vi "Get Variant Attributes.vi"(8 "错误输入":errorcluster, 11 "Variant":variant) -> (0 "错误输出":errorcluster, 1 "Values":variant[](array[variant]), 2 "Names":string[](array[string]), 3 "dup Variant":variant)   [LabVIEW 2012, in "TD Tools.lvlib"]
uses:
  TD Tools.lvlib
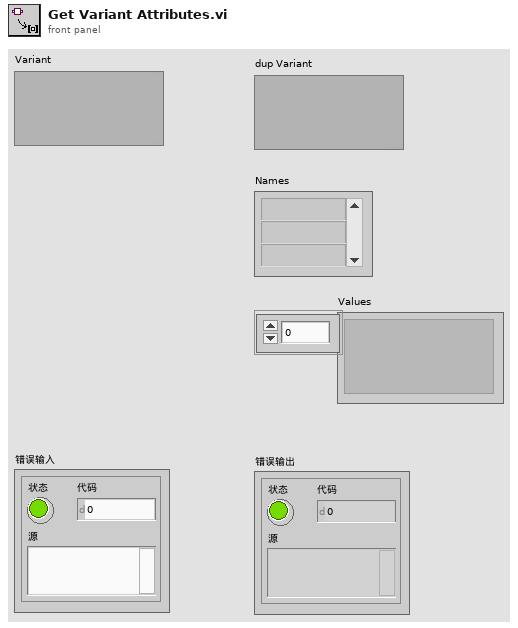
[diagram p1: front panel]
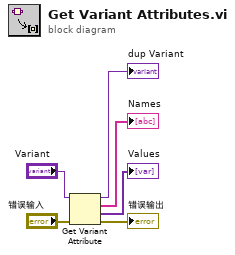
[diagram p0: block diagram]
diagram:
  n1 = Get Variant Attribute(Variant="Variant", error in="错误输入") -> (duplicate Variant=→"dup Variant":variant, names=→"Names":string[], values=→"Values":variant[], error out=→"错误输出":errorcluster)  [unwired: 2 in]
